vi "draw_manip_3d.vi"(8 "theta angle (deg)":dbl, 10 "gamma angle (deg)":dbl, 11 "manip tip coords":dbl[](array[numeric])) -> (3 "manip 3d location":dbl[][](array[numeric]))   [LabVIEW 2015]
uses:
  <vilib>/Analysis/NI_AALPro.lvlib
  <vilib>/Analysis/coordinate.llb/2D Cartesian Coordinate Rotation (Array).vi
  <vilib>/Analysis/coordinate.llb/2D Cartesian Coordinate Shift (Array).vi
panel:
  out "XY Graph":cluster{dbl[], dbl[]}(graph)
  in  "dy":dbl=2208.0 format="%#_13g"
  in  "dx":dbl=9100.0 format="%#_13g"
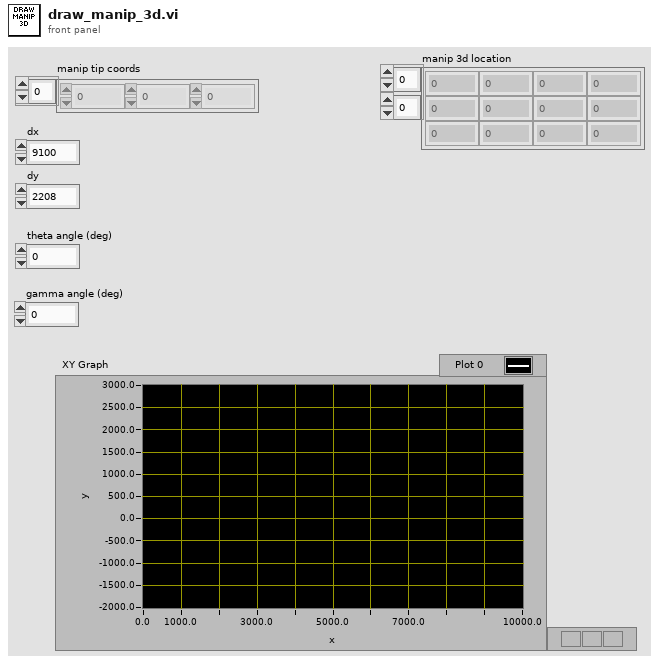
[diagram p1: front panel]
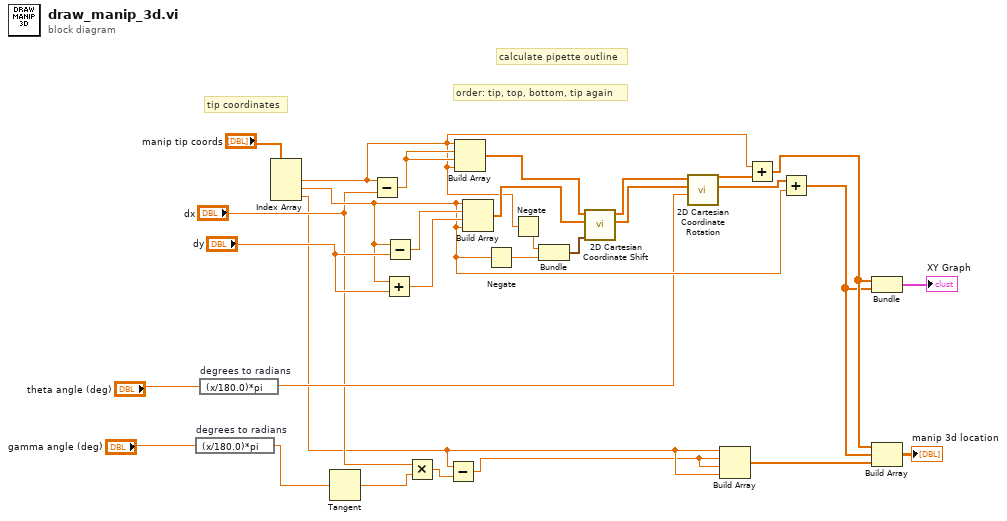
[diagram p0: block diagram]
diagram:
  # "order: tip, top, bottom, tip again"
  # "calculate pipette outline"
  # "tip coordinates"
  n1 = expression code="(x/180.0)*pi" "degrees to radians"("gamma angle (deg)") -> (w10:dbl)
  n2 = expression code="(x/180.0)*pi" "degrees to radians"("theta angle (deg)") -> (w12:dbl)
  n3 = Index Array(array="manip tip coords") -> (element #1=w17:dbl, element #2=w16:dbl, element #3=w6:dbl)  [unwired: 3 in]
  n4 = Tangent(1:w10) -> (0:w8:dbl)
  n5 = Subtract(x=w17, y="dx") -> (x-y=w29:dbl)
  n6 = Add(x=w16, y="dy") -> (x+y=w26:dbl)
  n7 = Subtract(x=w16, y="dy") -> (x-y=w27:dbl)
  n8 = Multiply(x="dx", y=w8) -> (x*y=w7:dbl)
  n9 = Subtract(x=w6, y=w7) -> (x-y=w5:dbl)
  n10 = Build Array(w17, w29, w29, w17) -> (w24:dbl[])
  n11 = Build Array(w16, w27, w26, w16) -> (w23:dbl[])
  n12 = Negate(x=w16) -> (-x=w20:dbl)
  n13 = Negate(x=w17) -> (-x=w19:dbl)
  n14 = Bundle(w19, w20) -> (w25:cluster{dbl, dbl})  [unwired: 1 in]
  n15 = call-poly <vilib>:"2D Cartesian Coordinate Shift.vi"("shift"=w25, "Y"=w23, "X"=w24) -> ("Y Out"=w21:dbl[], "X Out"=w22:dbl[])  [unwired: 6 in, 1 out]
  n16 = call-poly <vilib>:"2D Cartesian Coordinate Rotation.vi"("theta"=w12, "Y"=w21, "X"=w22) -> ("Y Out"=w15:dbl[], "X Out"=w18:dbl[])  [unwired: 6 in, 1 out]
  n17 = Build Array(w6, w5, w5, w6) -> (w2:dbl[])
  n18 = Add(x=w17, y=w18) -> (x+y=w4:dbl[])
  n19 = Add(x=w15, y=w16) -> (x+y=w3:dbl[])
  n20 = Bundle(w4, w3) -> (→"XY Graph":cluster{dbl[], dbl[]})  [unwired: 1 in]
  n21 = Build Array(w4, w3, w2) -> (→"manip 3d location":dbl[][])
